vi "velocity-unit-subvi-v2-k1.vi"(0 "Input":dbl, 1 "Unit":T1(ring)) -> (2 "output in counts":dbl, 3 "Unit":T1(ring), 4 "unit":string, 5 "Length and Unit":string)   [LabVIEW 2009]
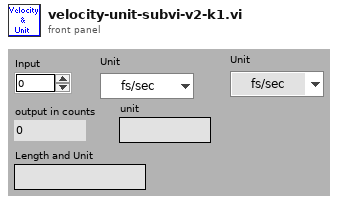
[diagram p1: front panel]
types:
  T1 = enum16{"fs/sec", "ps/sec", "um/sec", "mm/sec", "counts/sec"}
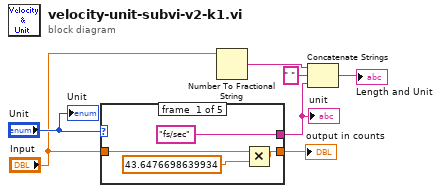
[diagram p0: block diagram]
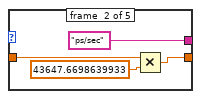
[diagram p2: hidden frame]
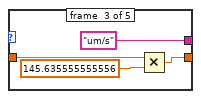
[diagram p3: hidden frame]
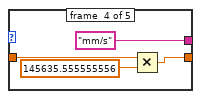
[diagram p4: hidden frame]
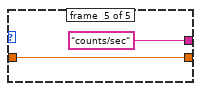
[diagram p5: hidden frame]
diagram:
  n1 = case shown="\"counts/sec\"" "Unit" {
    tunnel: "Input" -> [w11 w14 w17 w22 w25]
    tunnel: [w10 w13 w18 w21 w25] -> w6
    tunnel: ["fs/sec" "ps/sec" "um/s" "mm/s" "counts/sec"] -> w1
    frame #0 {
      n2 = Multiply(x=w11, y=43.6476698639934) -> (x*y=w10:dbl)
    }
    frame #1 {
      n3 = Multiply(x=w14, y=43647.6698639933) -> (x*y=w13:dbl)
    }
    frame #2 {
      n4 = Multiply(x=w17, y=145.635555555556) -> (x*y=w18:dbl)
    }
    frame #3 {
      n5 = Multiply(x=w22, y=145635.555555556) -> (x*y=w21:dbl)
    }
    frame #4 {
    }
  }
  "output in counts" <- w6
  "unit" <- w1
  n6 = Number To Fractional String(number="Input") -> (F-format string=w5:string)  [unwired: 3 in]
  n7 = Concatenate Strings(w5, " " ("string"), w1) -> (→"Length and Unit":string)
  "Unit" <- "Unit"
